vi "1 Tap 10-Bit.vi"() -> (0 "Pixels":cluster{"Pixel 0":u16})   [LabVIEW 2013]
uses:
  <vilib>/rvi/eio/common/nirviEmuTemplateMethod_errors.vi
  <vilib>/eio/EIONode/EIONode.xnode
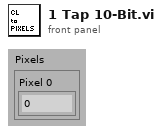
[diagram p1: front panel]
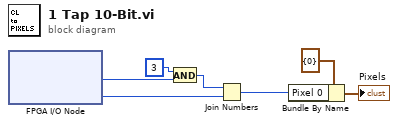
[diagram p0: block diagram]
diagram:
  n1 = xnode "FPGA I/O Node"() -> ("CL Port B"=w5:u8, "CL Port A"=w4:u8)  [unwired: 2 in, 2 out]
  n2 = And(x=u8 3 ("hi"), y=w5) -> (x .and. y?=w6:u8)
  n3 = Join Numbers(hi=w6, lo=w4) -> ((hi.lo)=w3:u16)
  n4 = Bundle By Name(cluster=cluster{"Pixel 0":u16} {"Pixel 0"=0} ("Data"), "Pixel 0"=w3) -> (→"Pixels":cluster{"Pixel 0":u16})
